vi "nufern common operation test 1.vi"() -> ()   [LabVIEW 2016]
uses:
  Common Operation Control 1.ctl
  Logistics Control 2.ctl
  Extended Operation Control 3.ctl
  Calibration Control.ctl
  <vilib>/Instr/_visa.llb/VISA Configure Serial Port (Instr).vi
panel:
  out "loop":i32
  out "read buffer":string
  in  "stop":bool
  in  "Enabled 2":bool
  in  "Enabled":bool
  out "string to crc":string
  out "CRC2":i32 format="0x%x"
  out "concatenated string":string
  in  "PAPA Address":i8=1 format="0x%02x"
  in  "Calibration":T1=128 format="0x%x" items=["Set Photodiode Threshold"=128, "Get All Photodiode Thresholds"=129, "Set Photodiode Trimpot Setpoint"=130, "Get All Photodiode Trimpot Setpoints"=131, "Set Preamp Pump Current Setpoint"=132, "Get All Preamp Pump Current Setpoints"=133, "Set Temperature Sensor Warning Threshold"=134, "Get Temperature Sensor Warning Threshold"=135, "Set Temperature Sensor Fault Threshold"=136, "Get Temperature Sensor Fault Threshold"=137, "Set HPE Photodiode Auto Threshold Delay"=138, "Get HPE Photodiode Auto Threshold Delay"=139]
  in  "Extended Operation":T2=67 format="0x%x" items=["Set HPE Photodiode Signal Drop Tolerance"=67, "Get HPE Photodiode Signal Drop Tolerance"=68, "Switch HPE Photodiode Fault Enable"=69, "Get Temperature Sensor Status"=70, "Switch Communication Timeout Enable"=71]
  in  "Logistics":T3=65 format="0x%x" items=["Set RS-485 Address"=65, "Get RS-485 Address"=66]
  in  "Common Operation":T4=4 format="0x%d" items=["Undefined", "Query: Get Unit Information", "Cmd: Emission On", "Cmd: Emission Off", "Query: Get Basic Status", "Query: Get Core Status", "Query: Get Extended Status", "Cmd: Clear Faults", "Cmd: Set Power Mode"]
  out "error out":errorcluster
  in  "error in (no error)":errorcluster
  in  "baud rate (9600)":u32=115200
  in  "VISA resource name":refnum<visa-resource-name>
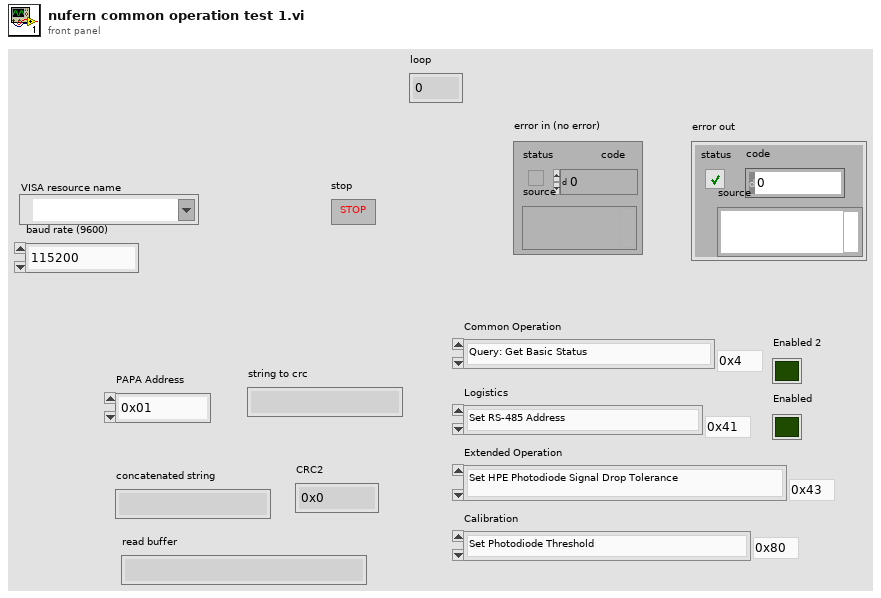
[diagram p1: front panel]
types:
  T1 = typedef "Calibration Control.ctl" = u16
  T2 = typedef "Extended Operation Control 3.ctl" = u16
  T3 = typedef "Logistics Control 2.ctl" = u16
  T4 = typedef "Common Operation Control 1.ctl" = u16
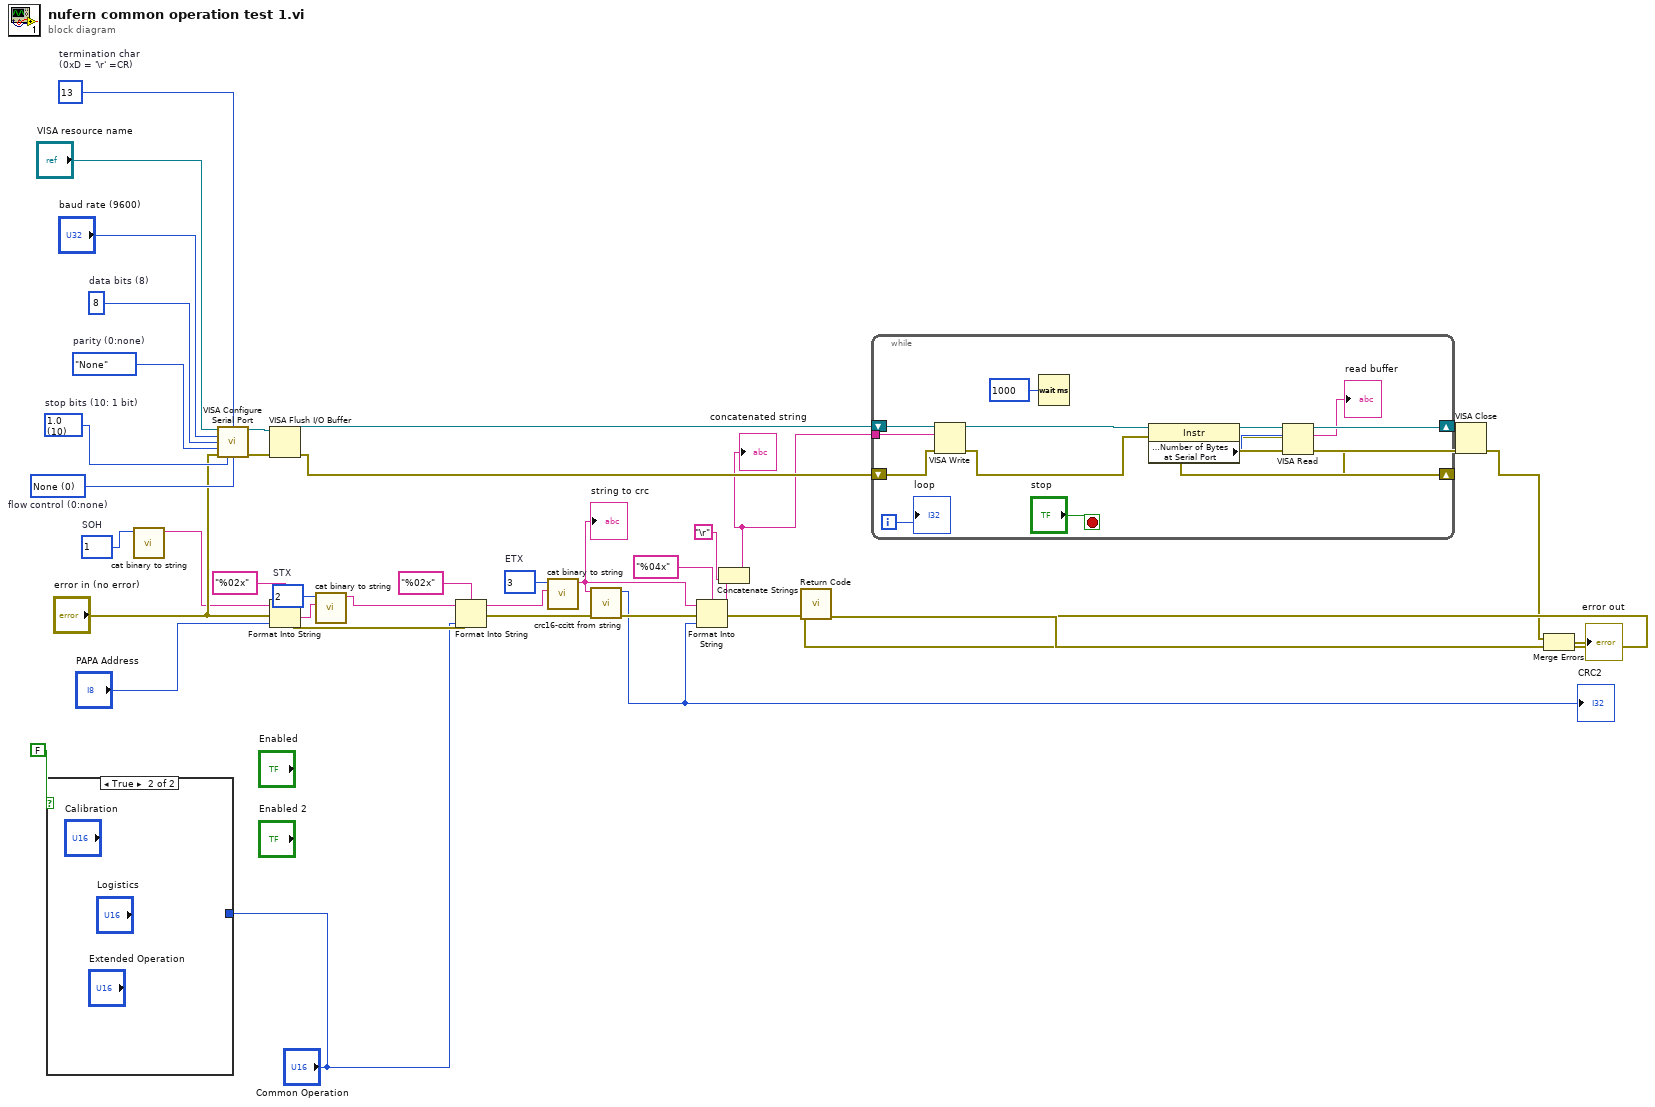
[diagram p0: block diagram]
diagram:
  w30 = u8 13  # termination char (0xD = '\r' =CR)
  w22 = 3  # ETX
  w15 = 2  # STX
  w13 = 1  # SOH
  w34 = u16 0 items=["None", "XON/XOFF", "RTS/CTS", "XON/XOFF & RTS/CTS", "DTR/DSR", "XON/XOFF & DTR/DSR"]  # flow control (0:none)
  w35 = u16 10 items=["1.0"=10, "1.5"=15, "2.0"=20]  # stop bits (10: 1 bit)
  w36 = enum16{"None", "Odd", "Even", "Mark", "Space"}."None"  # parity (0:none)
  w37 = u16 8  # data bits (8)
  n1 = case shown="True" FALSE ("Boolean") {
    tunnel: "Common Operation" -> [_ _]
    frame False {
    }
    frame True {
    }
  }
  n2 = call "cat binary to string.vi"("ETX"=w13) -> ("String out"=w12:string)  [unwired: 10 in]
  n3 = call-poly "VISA Configure Serial Port"("VISA resource name"="VISA resource name", "termination char\n(0xA = '\\n' = LF)"=w30, "baud rate (9600)"="baud rate (9600)", "data bits (8)"=w37, "parity (0:none)"=w36, "error in (no error)"="error in (no error)", "stop bits (10: 1 bit)"=w35, "flow control (0:none)"=w34) -> ("VISA resource name out"=w32:refnum<visa-resource-name>, "error out"=w33:errorcluster)  [unwired: 6 in]
  n4 = VISA Flush I/O Buffer(VISA resource name=w32, error in (no error)=w33) -> (VISA resource name out=w9:refnum<visa-resource-name>, error out=w7:errorcluster)  [unwired: 1 in]
  n5 = Format Into String(format string="%02x", initial string=w12, error in="error in (no error)", "PAPA Address") -> (resulting string=w16:string, error out=w18:errorcluster)
  n6 = call "cat binary to string.vi"("String in"=w16, "ETX"=w15) -> ("String out"=w14:string)  [unwired: 9 in]
  n7 = Format Into String(format string="%02x", initial string=w14, error in=w18, "Common Operation") -> (resulting string=w23:string, error out=w21:errorcluster)
  n8 = call "cat binary to string.vi"("String in"=w23, "ETX"=w22) -> ("String out"=w10:string)  [unwired: 9 in]
  "string to crc" <- w10
  n9 = call "crc16-ccitt from string.vi"("error in (no error)"=w21, "String"=w10) -> ("error out"=w20:errorcluster, "CRC Out"=w19:i32)  [unwired: 8 in]
  "CRC2" <- w19
  n10 = Format Into String(format string="%04x", initial string=w10, error in=w20, w19) -> (resulting string=w4:string, error out=w24:errorcluster)
  n11 = Concatenate Strings(w4, "\r") -> (w3:string)
  "concatenated string" <- w3
  n12 = call "Return Code.vi"("error in (no error)"=w24) -> ("error out"=w31:errorcluster)  [unwired: 9 in, 1 out]
  n13 = while {
    tunnel: w3 -> [w51]
    shift-right: [w46] -> w8
    shift-left: w9 -> [w53]
    shift-right: [w42] -> w6
    shift-left: w7 -> [w52]
    i -> [w40]
    stop <- "stop" stop-if-true
    n14 = VISA Write(VISA resource name=w53, write buffer=w51, error in (no error)=w52) -> (VISA resource name out=w48:refnum<visa-resource-name>, error out=w43:errorcluster)  [unwired: 1 out]
    n15 = Wait (ms)(milliseconds to wait=u32 1000) -> ()  [unwired: 1 out]
    n16 = property class="Instr"(reference=w48, error in=w43) -> (reference out=w47:refnum<visa-resource-name>, error out=w44:errorcluster, "Serial Settings:Number of Bytes at Serial Port"=w45:u32)
    n17 = VISA Read(VISA resource name=w47, byte count=w45, error in (no error)=w44) -> (VISA resource name out=w46:refnum<visa-resource-name>, read buffer=→"read buffer":string, error out=w42:errorcluster)  [unwired: 1 out]
    "loop" <- w40
  }
  n18 = VISA Close(VISA resource name=w8, error in (no error)=w6) -> (error out=w5:errorcluster)
  n19 = Merge Errors(w5, w31) -> (→"error out":errorcluster)
